vi "Dual Channel Log with Prompt Cancellation Handling.vi"() -> ()   [LabVIEW 2012]
doc: "This VI acquires temperature values every second and maintains a running average of the last five temperature measurements. This VI displays and logs both the raw data and the running average."
uses:
  File Operation.ctl
panel:
  in  "Stop Button":bool
  out "Temperature History":cluster{dbl, "Temperature Value":dbl}(graph)
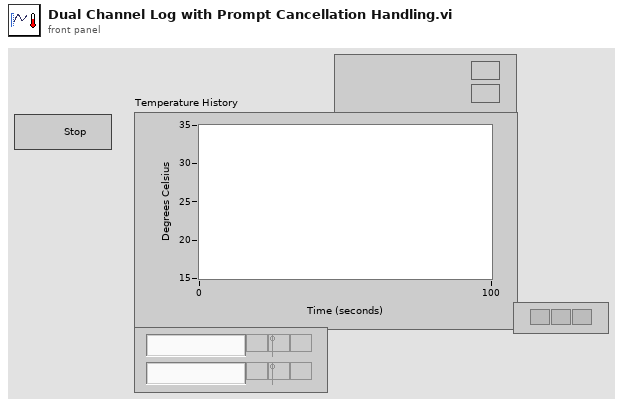
[diagram p1: front panel]
types:
  T1 = enum16{"open", "replace", "create", "open or create", "replace or create", "replace or create with confirmation"}
  T2 = typedef "File Operation.ctl" = enum16{"Prompt User", "Write Data", "No Write"}
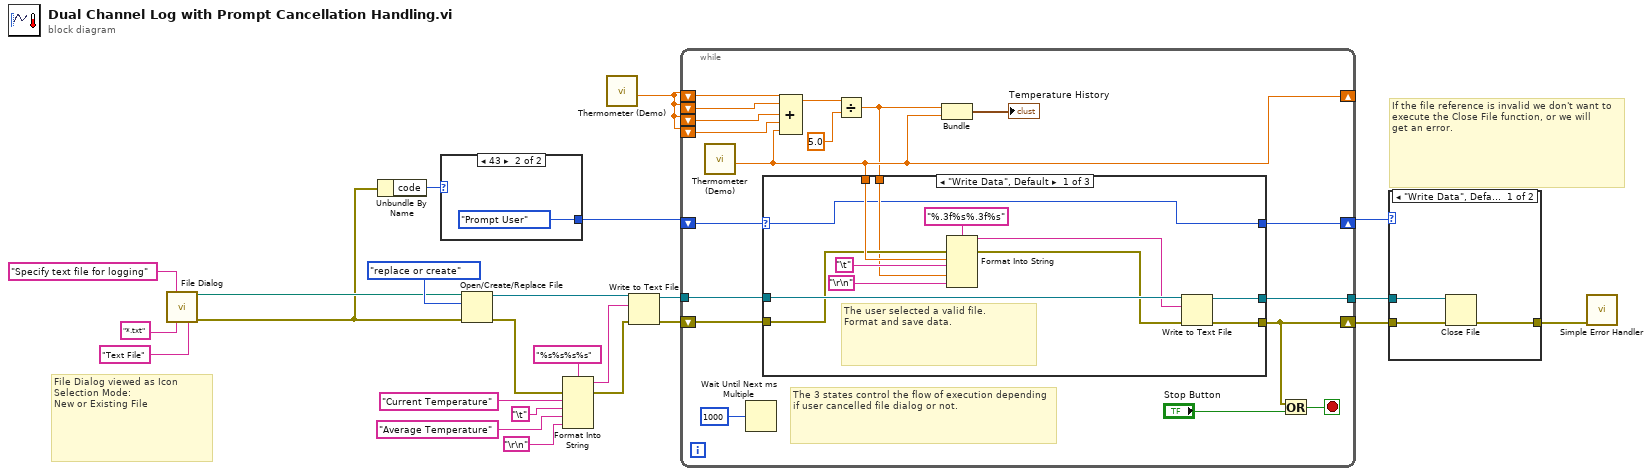
[diagram p0: block diagram]
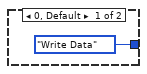
[diagram p3: hidden frame]
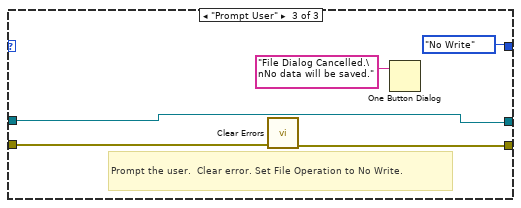
[diagram p5: hidden frame]
diagram:
  # "If the file reference is invalid we don't want to execute the Close File function, or we will\nget an error."
  # "File Dialog viewed as Icon\nSelection Mode:\nNew or Existing File"
  n1 = call "File Dialog"("prompt"="Specify text file for logging" ("pattern label"), "pattern (all files)"="*.txt", "pattern label"="Text File") -> ("selected path"=w18:path, "error out"=w4:errorcluster)  [unwired: 9 in, 2 out]
  n2 = Unbundle By Name(w4) -> ("code"=w5:i32)
  n3 = case shown="43" w5 {
    tunnel: [File_Operation."Write Data" ("Enum") File_Operation."Prompt User" ("Enum")] -> w3
    frame 0, Default {
    }
    frame 43 {
    }
  }
  n4 = Open/Create/Replace File(file path (use dialog)=w18, error in=w4, operation (0:open)=T1."replace or create") -> (refnum out=w19:refnum<file>, error out=w7:errorcluster)  [unwired: 4 out]
  n5 = Format Into String(format string="%s%s%s%s", error in=w7, "Current Temperature" ("string"), "\t", "Average Temperature" ("string"), "\r\n" ("End of Line Constant")) -> (resulting string=w8:string, error out=w6:errorcluster)  [unwired: 1 in]
  n6 = call "Thermometer (Demo).vi"() -> ("Temperature Value"=w24:dbl)  [unwired: 11 in]
  n7 = Write to Text File(file (use dialog)=w19, text=w8, error in=w6) -> (refnum out=w15:refnum<file>, error out=w14:errorcluster)  [unwired: 2 out]
  n8 = while {
    shift-right: [w31] -> _
    shift-left: w24 -> [w43]
    shift-left: w24 -> [w42]
    shift-left: w24 -> [w39]
    shift-left: w24 -> [w38]
    tunnel: w15 -> [w36]
    tunnel: [w35] -> w21
    shift-right: [w27] -> w2
    shift-left: w3 -> [w28]
    shift-right: [w34] -> w22
    shift-left: w14 -> [w30]
    stop <- w32 stop-if-true
    # "The 3 states control the flow of execution depending if user cancelled file dialog or not."
    n9 = call "Thermometer (Demo).vi"() -> ("Temperature Value"=w31:dbl)  [unwired: 11 in]
    n10 = Wait Until Next ms Multiple(millisecond multiple=u32 1000) -> ()  [unwired: 1 out]
    n11 = Compound Arithmetic op=ADD(w43, w42, w39, w38, w31) -> (w41:dbl)
    n12 = Divide(x=w41, y=5.0) -> (x/y=w29:dbl)
    n13 = case shown="\"Write Data\", Default" w28 {
      selector: w28 -> [w45 w59 _]
      tunnel: w36 -> [w56 w58 w61]
      tunnel: [w55 w58 w61] -> w35
      tunnel: [w54 w57 w62] -> w34
      tunnel: w31 -> [w53 _ _]
      tunnel: w30 -> [w51 w57 w63]
      tunnel: w29 -> [w46 _ _]
      tunnel: [w45 w59 File_Operation."No Write" ("Enum")] -> w27
      frame "Write Data", Default {
        # "The user selected a valid file. \nFormat and save data."
        n14 = Format Into String(format string="%.3f%s%.3f%s", error in=w51, w53, "\t", w46, "\r\n") -> (resulting string=w52:string, error out=w50:errorcluster)  [unwired: 1 in]
        n15 = Write to Text File(file (use dialog)=w56, text=w52, error in=w50) -> (refnum out=w55:refnum<file>, error out=w54:errorcluster)  [unwired: 2 out]
      }
      frame "No Write" {
        # "Execute the program, but don't save any data"
      }
      frame "Prompt User" {
        # "Prompt the user.  Clear error. Set File Operation to No Write."
        n16 = call <vilib>:"Clear Errors.vi"("error in (no error)"=w63) -> ("error out"=w62:errorcluster)  [unwired: 5 in, 1 out]
        n17 = One Button Dialog(message="File Dialog Cancelled.\nNo data will be saved.") -> ()  [unwired: 1 in, 1 out]
      }
    }
    n18 = Bundle(w29, "Temperature Value"=w31) -> (→"Temperature History":cluster{dbl, "Temperature Value":dbl})  [unwired: 1 in]
    n19 = Or(x=w34, y="Stop Button") -> (x .or. y?=w32:bool)
  }
  n20 = case shown="\"Write Data\", Default" w2 {
    tunnel: [w67 w68] -> w23
    tunnel: w22 -> [w66 w68]
    tunnel: w21 -> [w65 _]
    frame "Write Data", Default {
      n21 = Close File(refnum=w65, error in=w66) -> (error out=w67:errorcluster)  [unwired: 1 out]
    }
    frame "No Write" {
    }
  }
  n22 = call <vilib>:"Simple Error Handler.vi"("error in (no error)"=w23) -> ()  [unwired: 1 in, 8 out]
